vi "Get CD Drive.vi"() -> (0 "CD path":path)   [LabVIEW 2011]
uses:
  KERNEL32.DLL
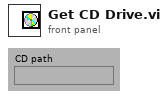
[diagram p1: front panel]
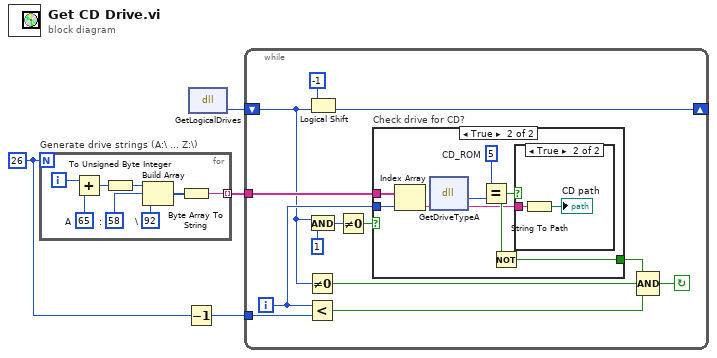
[diagram p0: block diagram]
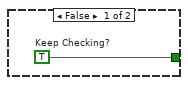
[diagram p2: hidden frame]
diagram:
  w3 = 26
  n1 = for "Generate drive strings (A:\\ ... Z:\\)" {
    N: w3 -> [_]
    tunnel: [w5] -> w4 mode=indexing
    i -> [w12]
    w7 = u8 92  # \
    w8 = u8 58  # :
    w11 = 65  # A
    n2 = Add(x=w12, y=w11) -> (x+y=w10:i32)
    n3 = To Unsigned Byte Integer(number=w10) -> (unsigned 8bit integer=w9:u8)
    n4 = Build Array(w9, w8, w7) -> (w6:u8[])
    n5 = Byte Array To String(unsigned byte array=w6) -> (string=w5:string)
  }
  n6 = Decrement(x=w3) -> (x-1=w2:i32)
  n7 = dll-call lib="KERNEL32.DLL" fn="GetLogicalDrives"() -> ("drive_flags"=w1:i32)  [unwired: 3 in, 2 out]
  n8 = while {
    shift-right: [w23] -> _
    shift-left: w1 -> [w14]
    tunnel: w4 -> [w22]
    tunnel: w2 -> [w25]
    i -> [w21]
    stop <- w16 continue-if-true
    n9 = Not Equal To 0?(x=w14) -> (x != 0?=w17:bool)
    n10 = Less?(x=w21, y=w25) -> (x < y?=w18:bool)
    n11 = Logical Shift(y=-1, x=w14) -> (x << y=w23:i32)
    n12 = And(x=w14, y=1) -> (x .and. y?=w20:i32)
    n13 = Not Equal To 0?(x=w20) -> (x != 0?=w19:bool)
    n14 = case "Check drive for CD?" shown="True" w19 {
      tunnel: w22 -> [_ w34]
      tunnel: w21 -> [_ w33]
      tunnel: [w26 w29] -> w15
      frame False {
        w26 = TRUE  # Keep Checking?
      }
      frame True {
        w28 = 5  # CD_ROM
        n15 = Index Array(array=w34, index=w33) -> (element=w32:string)
        n16 = dll-call lib="KERNEL32.DLL" fn="GetDriveTypeA" label="GetDriveType"("nDrive"=w32) -> ("drive_type"=w31:i32, "nDrive"=w27:string)  [unwired: 3 in, 2 out]
        n17 = Equal?(x=w28, y=w31) -> (x = y?=w30:bool)
        n18 = Not(x=w30) -> (.not. x?=w29:bool)
        n19 = case shown="True" w30 {
          tunnel: w27 -> [_ w36]
          frame False {
          }
          frame True {
            n20 = String To Path(string=w36) -> (path=→"CD path":path)
          }
        }
      }
    }
    n21 = Compound Arithmetic op=AND(w15, w17, w18) -> (w16:bool)
  }
